vi "Get_measurement_samplingdata.vi"(0 "SPU":refnum<k24>, 1 "STSProcess.ILSTS":refnum<k24>, 5 "Meas_monitor_struct":refnum<k24>[](array[refnum]), 7 "MPM":refnum<k24>[](array[refnum]), 9 "Data_struct":refnum<k24>[](array[refnum]), 11 "错误输入（无错误）":errorcluster, 12 "SweepCount":i32) -> (15 "error out":errorcluster)   [LabVIEW 2017]
doc: "Get logging measurement data & add in"
uses:
  D:/test/ILSTS/LV_IL_Sample/DLL/STSProcess.dll
  DLL/STSProcess.dll
  D:/test/ILSTS/LV_IL_Sample/DLL/InstrumentDLL.dll
  DLL/InstrumentDLL.dll
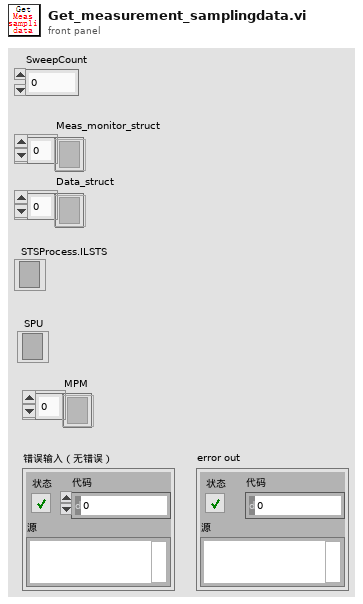
[diagram p1: front panel]
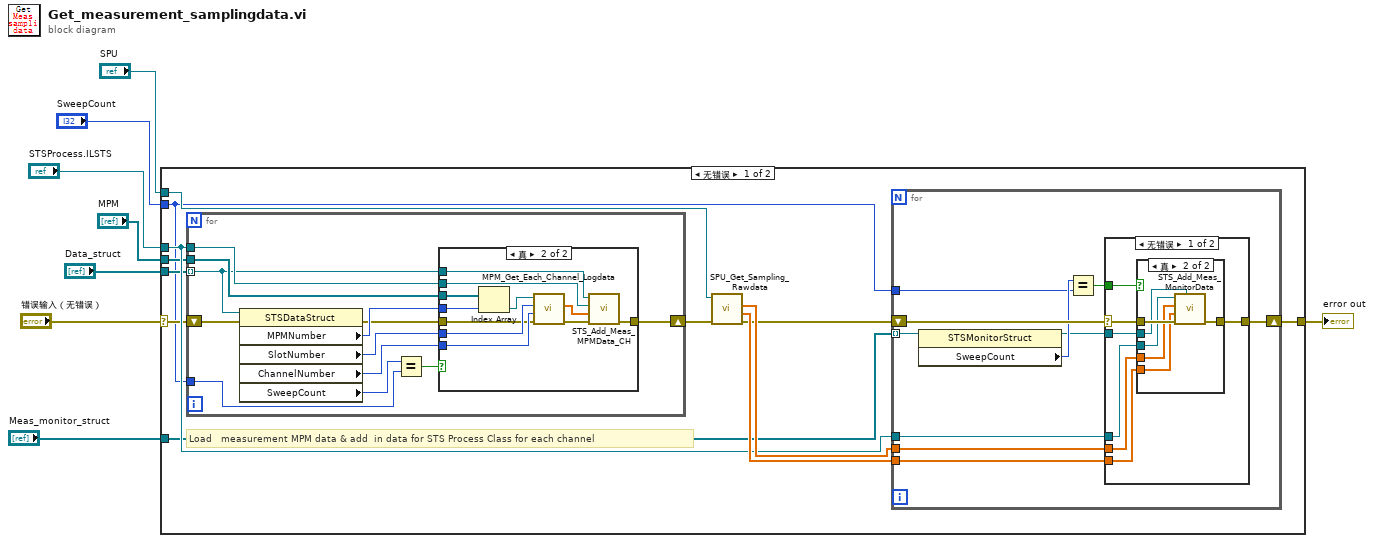
[diagram p0: block diagram]
diagram:
  n1 = case shown="无错误" "错误输入（无错误）" {
    selector: "错误输入（无错误）" -> [w11 w70]
    tunnel: "STSProcess.ILSTS" -> [w18 _]
    tunnel: "Meas_monitor_struct" -> [w17 _]
    tunnel: "SPU" -> [w16 _]
    tunnel: "MPM" -> [w14 _]
    tunnel: "Data_struct" -> [w13 _]
    tunnel: [w12 w70] -> w5
    tunnel: "SweepCount" -> [w10 _]
    frame No Error {
      # "Load　measurement MPM data & add  in data for STS Process Class for each channel"
      n2 = for {
        tunnel: w13 -> [w49] mode=indexing
        tunnel: w14 -> [w55]
        tunnel: w18 -> [w50]
        tunnel: w10 -> [w47]
        shift-right: [w51] -> w15
        shift-left: w11 -> [w52]
        n3 = property on="属性节点" class="STSDataStruct"(reference=w49, error in=w52) -> (error out=w53:errorcluster, "MPMNumber"=w54:i32, "SlotNumber"=w57:i32, "ChannelNumber"=w56:i32, "SweepCount"=w48:i32)  [unwired: 1 out]
        n4 = Equal?(x=w48, y=w47) -> (x = y?=w46:bool)
        n5 = case shown="真" w46 {
          tunnel: w57 -> [_ w69]
          tunnel: w56 -> [_ w68]
          tunnel: w55 -> [_ w67]
          tunnel: w54 -> [_ w66]
          tunnel: w53 -> [w58 w65]
          tunnel: [w58 w63] -> w51
          tunnel: w50 -> [_ w60]
          tunnel: w49 -> [_ w59]
          frame False {
          }
          frame True {
            n6 = Index Array(array=w67, index=w66) -> (element=w64:refnum<k24>)
            n7 = call "MPM_Get_Each_Channel_Logdata.vi"("error in (no error)"=w65, "channelNumber"=w68, "moduleNumber"=w69, ".NET Reference in"=w64) -> ("error out"=w62:errorcluster, "data out"=w61:sgl[])  [unwired: 5 in, 1 out]
            n8 = call "STS_Add_Meas_MPMData_CH.vi"("错误输入（无错误）"=w62, "data"=w61, "STSProcess.ILSTS"=w60, ".NET引用句柄输入"=w59) -> ("错误输出"=w63:errorcluster)  [unwired: 6 in, 1 out]
          }
        }
      }
      n9 = call "SPU_Get_Sampling_Rawdata.vi"("错误输入（无错误）"=w15, "SPU"=w16) -> ("error out"=w9:errorcluster, "monitor"=w20:sgl[], "trigger"=w19:sgl[])  [unwired: 5 in, 1 out]
      n10 = for {
        tunnel: w17 -> [w25] mode=indexing
        tunnel: w18 -> [w30]
        tunnel: w19 -> [w29]
        tunnel: w20 -> [w28]
        shift-right: [w26] -> w12
        shift-left: w9 -> [w27]
        tunnel: w10 -> [w23]
        n11 = property on="属性节点" class="STSMonitorStruct"(reference=w25) -> (reference out=w21:refnum<k24>, "SweepCount"=w24:i32)  [unwired: 1 in, 1 out]
        n12 = Equal?(x=w24, y=w23) -> (x = y?=w22:bool)
        n13 = case shown="无错误" w27 {
          selector: w27 -> [w36 w45]
          tunnel: w30 -> [w35 _]
          tunnel: w21 -> [w32 _]
          tunnel: w29 -> [w34 _]
          tunnel: w28 -> [w33 _]
          tunnel: [w37 w45] -> w26
          tunnel: w22 -> [w31 _]
          frame No Error {
            n14 = case shown="真" w31 {
              tunnel: [w38 w44] -> w37
              tunnel: w36 -> [w38 w43]
              tunnel: w35 -> [_ w42]
              tunnel: w34 -> [_ w41]
              tunnel: w33 -> [_ w40]
              tunnel: w32 -> [_ w39]
              frame False {
              }
              frame True {
                n15 = call "STS_Add_Meas_MonitorData.vi"("setting"=w39, "错误输入（无错误）"=w43, "monitorData"=w40, "triggerIndex"=w41, "STSProcess.ILSTS"=w42) -> ("错误输出"=w44:errorcluster)  [unwired: 5 in, 1 out]
              }
            }
          }
          frame Error {
          }
        }
      }
    }
    frame Error {
    }
  }
  "error out" <- w5
